vi "TEST 2-dim swerve direction indicators.vi"() -> ()   [LabVIEW 2023]
panel:
  out "appended array":dbl[][](array[numeric])
  out "element":cluster{"row":i32, "col":i32}
  out "output array":dbl[][](array[numeric])
  in  "stop":bool
  in  "Dial 2":i8(knob) min=0 max=3 step=1 scale=0.0..3.0
  in  "Dial":dbl(knob) scale=0.0..360.0
  out "SWERVE ANGLES":dbl[][](array[knob]) scale=0.0..360.0
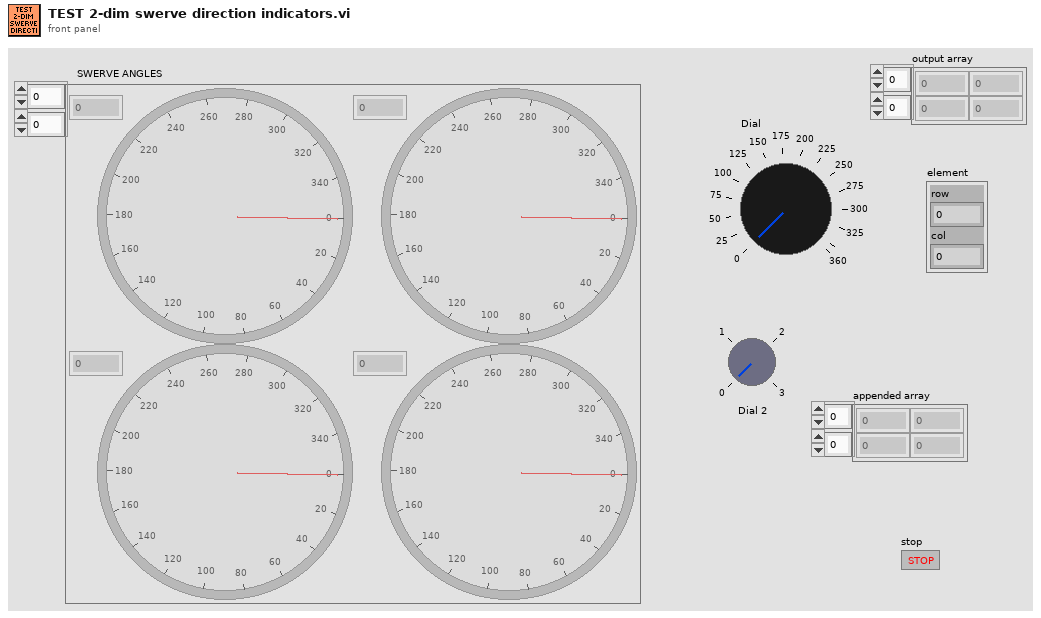
[diagram p1: front panel]
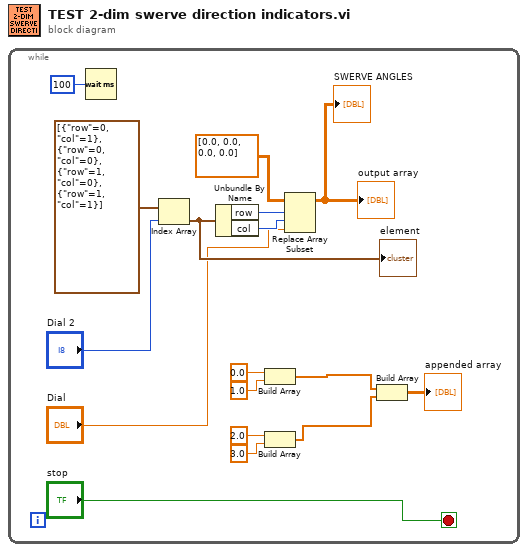
[diagram p0: block diagram]
diagram:
  n1 = while {
    stop <- "stop" stop-if-true
    n2 = Wait (ms)(milliseconds to wait=u32 100) -> ()  [unwired: 1 out]
    n3 = Index Array(array=cluster{"row":i32, "col":i32}[] [{"row"=0, "col"=1}, {"row"=0, "col"=0}, {"row"=1, "col"=0}, {"row"=1, "col"=1}], index="Dial 2") -> (element=w13:cluster{"row":i32, "col":i32})
    "element" <- w13
    n4 = Unbundle By Name(w13) -> ("row"=w12:i32, "col"=w11:i32)
    n5 = Build Array(0.0 ("element"), 1.0 ("element")) -> (w6:dbl[])
    n6 = Build Array(2.0 ("element"), 3.0 ("element")) -> (w1:dbl[])
    n7 = Replace Array Subset(array=dbl[][] [[0.0, 0.0], [0.0, 0.0]], new element="Dial", index (row)=w12, index (col)=w11) -> (→"SWERVE ANGLES" →"output array":dbl[][])
    n8 = Build Array(w6, w1) -> (→"appended array":dbl[][])
  }
